vi "write exposure time.vi"(11 "exposure time(ms)":dbl=1.0) -> (3 "Success":bool)   [LabVIEW 2018]
uses:
  Dll1_x64_191014_0/Dll1_x64_191014_0.lvlib
panel:
  out "spi":string[][](array[string])
  out "status":string
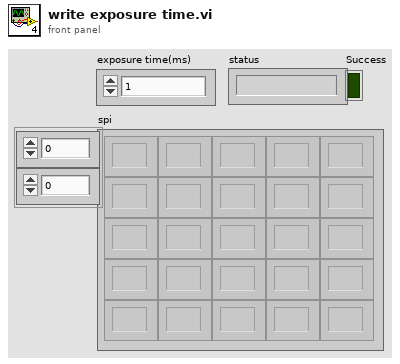
[diagram p1: front panel]
types:
  T1 = enum32{"invalid app kind", "Development System", "Run Time System", "Student Edition", "Embedded LabVIEW", "Evaluation", "Custom"}
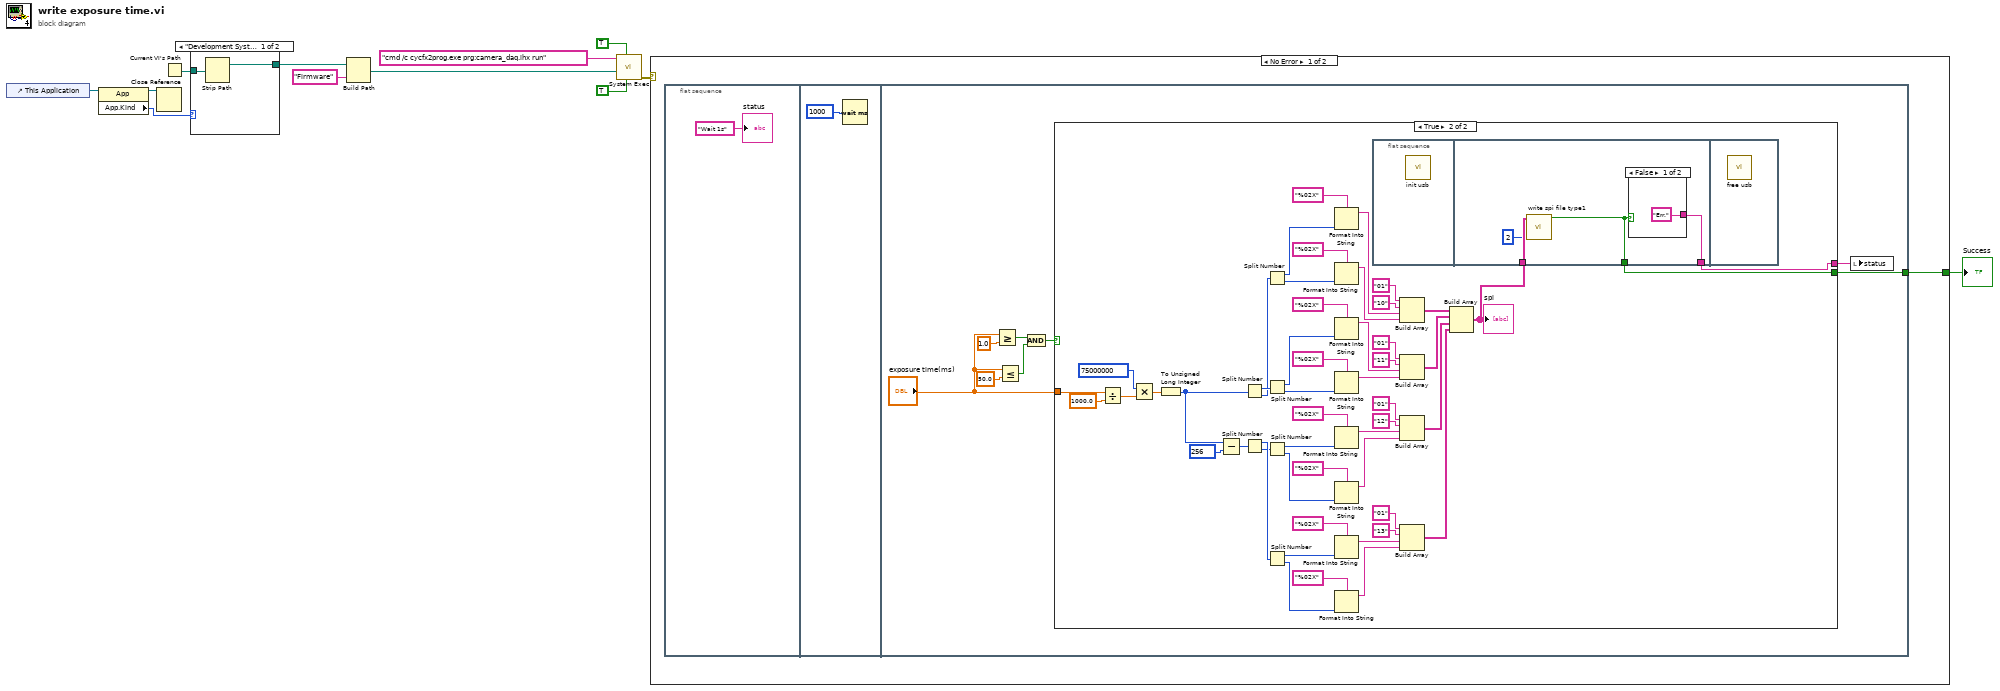
[diagram p0: block diagram]
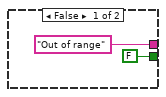
[diagram p2: hidden frame]
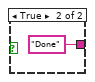
[diagram p3: hidden frame]
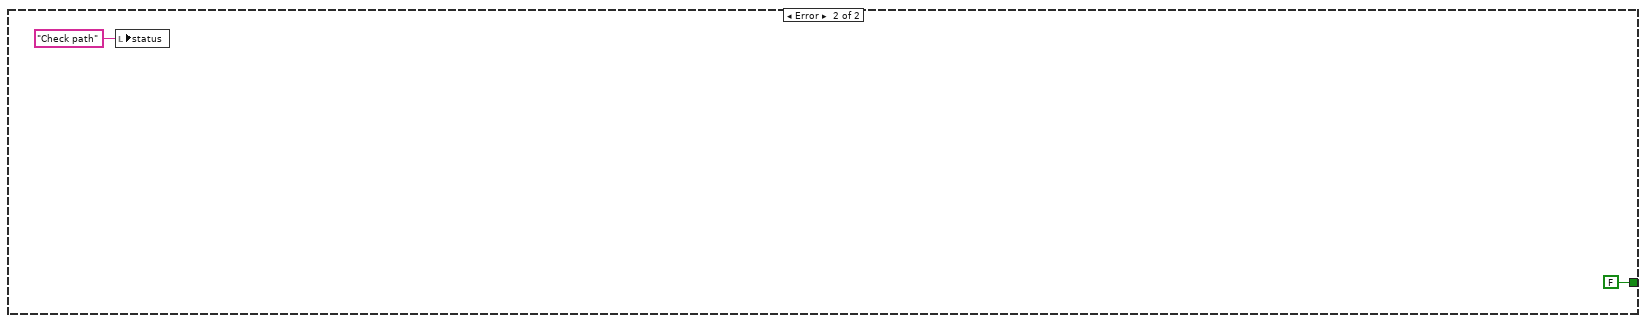
[diagram p4: hidden frame]
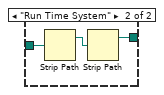
[diagram p5: hidden frame]
diagram:
  n1 = control-ref of="This Application"() -> (w9:refnum<vi>)
  n2 = property class="App"(reference=w9) -> (reference out=w10:refnum<vi>, "App.Kind"=w11:T1)  [unwired: 1 in, 1 out]
  n3 = Close Reference(reference=w10) -> ()  [unwired: 1 in, 1 out]
  n4 = Current VI's Path() -> (path=w12:path)
  n5 = case shown="\"Development System\", Default" w11 {
    tunnel: w12 -> [w14 w17]
    tunnel: [w13 w15] -> w8
    frame "Development System", Default {
      n6 = Strip Path(path=w14) -> (stripped path=w13:path)  [unwired: 1 out]
    }
    frame "Run Time System" {
      n7 = Strip Path(path=w17) -> (stripped path=w16:path)  [unwired: 1 out]
      n8 = Strip Path(path=w16) -> (stripped path=w15:path)  [unwired: 1 out]
    }
  }
  n9 = Build Path(base path=w8, name or relative path="Firmware") -> (appended path=w3:path)
  n10 = call <vilib>:"System Exec.vi"("run minimized? (F)"=TRUE, "wait until completion? (T)"=TRUE, "working directory"=w3, "command line"="cmd /c cycfx2prog.exe prg:camera_daq.ihx run") -> ("error out"=w1:errorcluster)  [unwired: 4 in, 3 out]
  n11 = case shown="No Error" w1 {
    tunnel: [w18 FALSE ("res")] -> w7
    frame No Error {
      n12 = flat-sequence {
        tunnel: [w21] -> w18
        frame #0 {
          "status" <- "Wait 1s" ("test status")
        }
        frame #1 {
          n13 = Wait (ms)(milliseconds to wait=u32 1000) -> ()  [unwired: 1 out]
        }
        frame #2 {
          n14 = Greater Or Equal?(x="exposure time(ms)", y=1.0) -> (x >= y?=w27:bool)
          n15 = Less Or Equal?(x="exposure time(ms)", y=50.0) -> (x <= y?=w26:bool)
          n16 = And(x=w27, y=w26) -> (x .and. y?=w23:bool)
          n17 = case shown="True" w23 {
            tunnel: "exposure time(ms)" -> [_ w35]
            tunnel: [FALSE ("res") w32] -> w21
            tunnel: ["Out of range" ("result") w31] -> w22
            frame False {
            }
            frame True {
              n18 = Divide(x=w35, y=1000.0) -> (x/y=w34:dbl)
              n19 = Multiply(x=75000000, y=w34) -> (x*y=w80:dbl)
              n20 = To Unsigned Long Integer(number=w80) -> (unsigned 32bit integer=w69:u32)
              n21 = Subtract(x=w69, y=u32 256) -> (x-y=w57:u32)
              n22 = Split Number(x=w69) -> (hi(x)=w79:u16, lo(x)=w78:u16)
              n23 = Split Number(x=w57) -> (hi(x)=w67:u16, lo(x)=w66:u16)
              n24 = Split Number(x=w78) -> (hi(x)=w71:u8, lo(x)=w70:u8)
              n25 = Split Number(x=w79) -> (hi(x)=w76:u8, lo(x)=w72:u8)
              n26 = Split Number(x=w66) -> (hi(x)=w59:u8, lo(x)=w58:u8)
              n27 = Split Number(x=w67) -> (hi(x)=w64:u8, lo(x)=w60:u8)
              n28 = Format Into String(format string="%02X", w71) -> (resulting string=w54:string)  [unwired: 2 in, 1 out]
              n29 = Format Into String(format string="%02X", w70) -> (resulting string=w53:string)  [unwired: 2 in, 1 out]
              n30 = Format Into String(format string="%02X", w76) -> (resulting string=w49:string)  [unwired: 2 in, 1 out]
              n31 = Format Into String(format string="%02X", w72) -> (resulting string=w48:string)  [unwired: 2 in, 1 out]
              n32 = Format Into String(format string="%02X", w59) -> (resulting string=w43:string)  [unwired: 2 in, 1 out]
              n33 = Format Into String(format string="%02X", w58) -> (resulting string=w42:string)  [unwired: 2 in, 1 out]
              n34 = Format Into String(format string="%02X", w64) -> (resulting string=w41:string)  [unwired: 2 in, 1 out]
              n35 = Format Into String(format string="%02X", w60) -> (resulting string=w40:string)  [unwired: 2 in, 1 out]
              n36 = flat-sequence {
                tunnel: w33 -> [w85]
                tunnel: [w84] -> w32
                tunnel: [w83] -> w31
                frame #0 {
                  n37 = call "init usb.vi"() -> ()  [unwired: 12 in]
                }
                frame #1 {
                  n38 = call "write spi file type1.vi"("milliseconds to wait"=u32 2, "addr/data"=w85) -> ("res"=w84:bool)  [unwired: 9 in]
                  n39 = case shown="False" w84 {
                    tunnel: ["Err." ("result") "Done" ("result")] -> w83
                    frame False {
                    }
                    frame True {
                    }
                  }
                }
                frame #2 {
                  n40 = call "free usb.vi"() -> ()  [unwired: 12 in]
                }
              }
              n41 = Build Array("01" ("string"), "10" ("string"), w54, w53) -> (w52:string[])
              n42 = Build Array("01" ("string"), "11" ("string"), w49, w48) -> (w39:string[])
              n43 = Build Array("01" ("string"), "12" ("string"), w43, w42) -> (w38:string[])
              n44 = Build Array("01" ("string"), "13" ("string"), w41, w40) -> (w37:string[])
              n45 = Build Array(w52, w39, w38, w37) -> (w33:string[][])
              "spi" <- w33
            }
          }
          n46 = local write "status"(w22) -> ()
        }
      }
    }
    frame Error {
      n47 = local write "status"("Check path" ("status")) -> ()
    }
  }
  "Success" <- w7
